vi "CLOSE.vi"(11 "Pump_1AI_1DO_2DI in":refnum<class "NeedleValve.lvclass">) -> (3 "Pump_1AI_1DO_2DI out":refnum<class "NeedleValve.lvclass">)   [LabVIEW 2019]
uses:
  TypeDef/Needle Valve State.ctl
  NeedleValve.lvclass
  D:/GIT H4000/H4000/src/Device_class/Device.lvclass
  D:/GIT H4000/H4000/src/Proccess_class/Proccess.lvclass
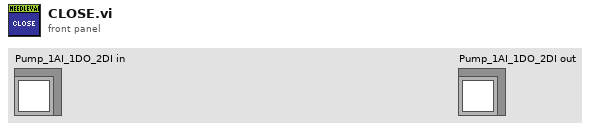
[diagram p1: front panel]
types:
  T1 = typedef "Needle Valve State.ctl" = enum16{"IDLE", "OPEN", "CLOSE", "OPENING", "CLOSING", "STOP"}
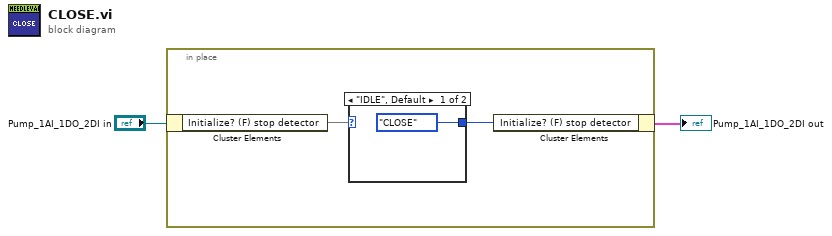
[diagram p0: block diagram]
diagram:
  n1 = in-place {
    n2 = in-place-cluster #1("Pump_1AI_1DO_2DI in") -> ("Initialize? (F) stop detector"=w3)
    n3 = case shown="\"IDLE\", Default" w3 {
      selector: w3 -> [_ w6]
      tunnel: [Needle_Valve_State."CLOSE" ("StateValveModbus") w6] -> w4
      frame "IDLE", Default {
      }
      frame "CLOSING" {
      }
    }
    n4 = in-place-cluster #1("Initialize? (F) stop detector"=w4) -> (→"Pump_1AI_1DO_2DI out":cluster{})
  }
